vi "SENS_AVER_STAT_ON_OFF.vi"(0 "VISA IN":refnum<visa-resource-name>, 1 "State":bool, 5 "error in":errorcluster, 7 "Channel":i32) -> (14 "VISA Out":refnum<visa-resource-name>, 19 "error out":errorcluster)   [LabVIEW 2018, in "PNA-X.lvlib"]
doc: "SENSe<cnum>:AVERage[:STATe] <ON | OFF> \n(Read-Write) Turns trace averaging ON or OFF. \nParameters \n<cnum> Any existing channel number; if unspecified, value is set to 1. \n<ON | OFF> ON (or 1) - turns averaging ON. \nOFF (or 0) - turns averaging OFF. \nExamples SENS:AVER ON \nsense2:average:state off \nQuery Syntax SENSe<cnum>:AVERage[:STATe]? \nReturn Type Boolean (1 = ON, 0 = OFF) \nDefault Off \n1620\n\nSense:Bandwidth Commands \nSee Also \nExample Programs \nLearn about IF Bandwidth \nSynchronizing the PNA and Controller \nSCPI Command Tree"
uses:
  PNA-X.lvlib
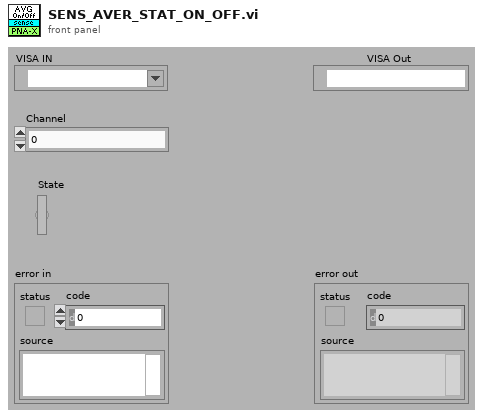
[diagram p1: front panel]
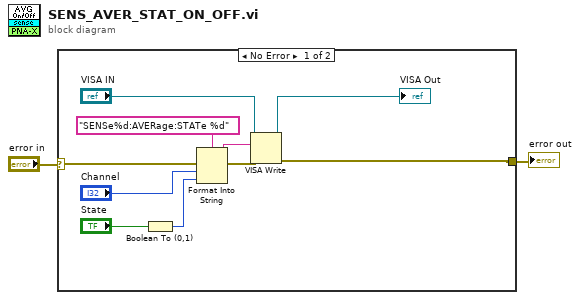
[diagram p0: block diagram]
diagram:
  n1 = case shown="No Error" "error in" {
    selector: "error in" -> [w12 w13]
    tunnel: [w8 w13] -> w1
    frame No Error {
      n2 = Boolean To (0,1)(Boolean="State") -> (0, 1=w4:i16)
      n3 = Format Into String(format string="SENSe%d:AVERage:STATe %d" ("Cmdline"), error in=w12, "Channel", w4) -> (resulting string=w10:string, error out=w11:errorcluster)  [unwired: 1 in]
      n4 = VISA Write(VISA resource name="VISA IN", write buffer=w10, error in (no error)=w11) -> (VISA resource name out=→"VISA Out":refnum<visa-resource-name>, error out=w8:errorcluster)  [unwired: 1 out]
    }
    frame Error {
    }
  }
  "error out" <- w1
